vi "followMotionProfile.vi"(9 "Constants":T1={"kV"=0.00542, "kA"=0.0008, "PV"=0.0, "PP"=0.0, "DV"=0.0}, 10 "Feedback":cluster{"accel":dbl, "vel":dbl, "pos":dbl}, 11 "Target":cluster{"accel":dbl, "vel":dbl, "pos":dbl}) -> (3 "Duty Cycle":dbl)   [LabVIEW 2015]
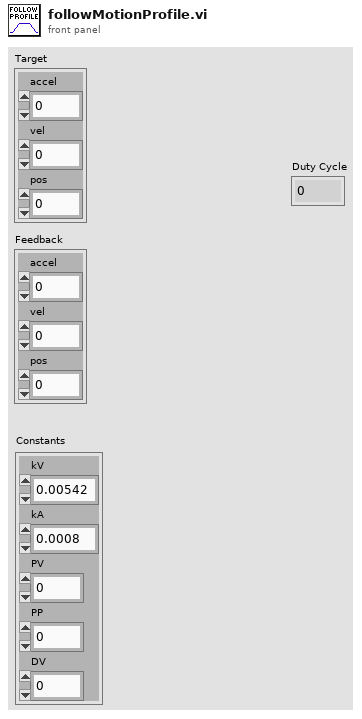
[diagram p1: front panel]
types:
  T1 = cluster{"kV":dbl, "kA":dbl, "PV":dbl, "PP":dbl, "DV":dbl}
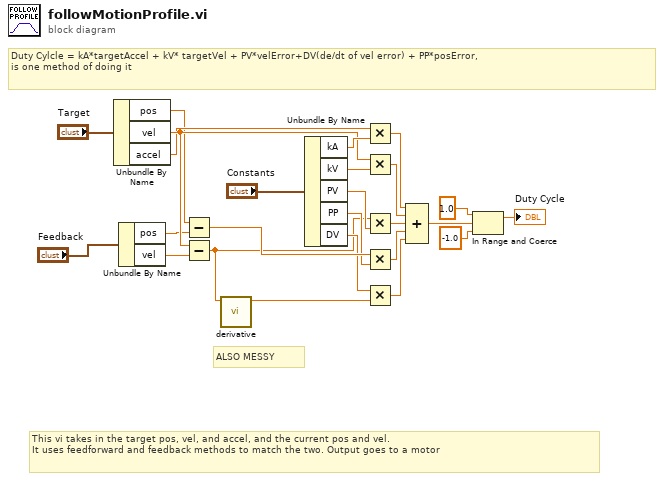
[diagram p0: block diagram]
diagram:
  # "This vi takes in the target pos, vel, and accel, and the current pos and vel.\nIt uses feedforward and feedback methods to match the two. Output goes to a motor"
  # "ALSO MESSY"
  # "Duty Cylcle = kA*targetAccel + kV* targetVel + PV*velError+DV(de/dt of vel error) + PP*posError,\nis one method of doing it"
  n1 = Unbundle By Name("Target") -> ("pos"=w3:dbl, "vel"=w6:dbl, "accel"=w5:dbl)
  n2 = Unbundle By Name("Feedback") -> ("pos"=w4:dbl, "vel"=w14:dbl)
  n3 = Subtract(x=w3, y=w4) -> (x-y=w11:dbl)
  n4 = Subtract(x=w6, y=w14) -> (x-y=w2:dbl)
  n5 = call "derivative.vi"("x"=w2) -> ("dx/dt"=w1:dbl)  [unwired: 10 in]
  n6 = Unbundle By Name("Constants") -> ("kA"=w23:dbl, "kV"=w22:dbl, "PV"=w13:dbl, "PP"=w10:dbl, "DV"=w8:dbl)
  n7 = Multiply(x=w5, y=w23) -> (x*y=w20:dbl)
  n8 = Multiply(x=w6, y=w22) -> (x*y=w21:dbl)
  n9 = Multiply(x=w2, y=w13) -> (x*y=w12:dbl)
  n10 = Multiply(x=w11, y=w10) -> (x*y=w9:dbl)
  n11 = Multiply(x=w8, y=w1) -> (x*y=w7:dbl)
  n12 = Compound Arithmetic op=ADD(w20, w21, w12, w9, w7) -> (w19:dbl)
  n13 = In Range and Coerce(upper limit=1.0, x=w19, lower limit=-1.0) -> (coerced(x)=→"Duty Cycle":dbl)  [unwired: 1 out]
